vi "Fire User Event - Stop Externo.vi"(8 "error in (no error)":errorcluster, 11 "Stop Externo":bool=TRUE) -> (0 "error out":errorcluster)   [LabVIEW 2019, in "User Events.lvlib"]
doc: "Send the Stop event to stop the Event Handling Loop."
uses:
  User Events.lvlib
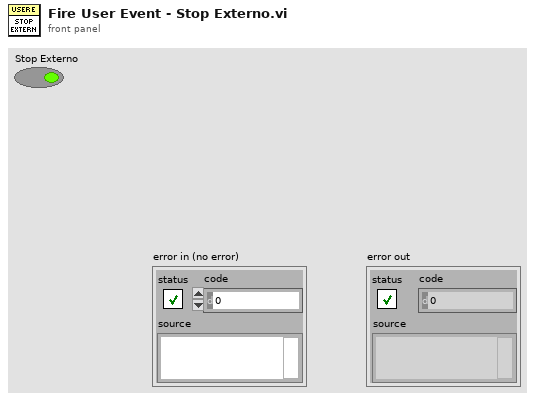
[diagram p1: front panel]
types:
  T1 = typedef "User Events.lvlib/User Events Typedef.ctl" = cluster{"Stop Event Interno":refnum<user-event>, "Volts":refnum<user-event>, "QMH Stop":refnum<user-event>, "Stop Event Externo":refnum<user-event>}
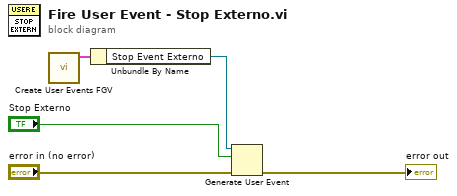
[diagram p0: block diagram]
diagram:
  n1 = call "Create User Events FGV.vi"() -> ("User Events"=w3:T1)  [unwired: 10 in, 1 out]
  n2 = Unbundle By Name(w3) -> ("Stop Event Externo"=w2:refnum<user-event>)
  n3 = Generate User Event(user event=w2, event data cluster="Stop Externo", error in="error in (no error)") -> (error out=→"error out":errorcluster)  [unwired: 1 in, 1 out]
